vi "Set Fill Color.vi"(8 "error in (no error)":errorcluster, 9 "Color":u32(colorbox), 10 "Shape refnum":refnum<k7>) -> (0 "error out":errorcluster, 2 "reference out":refnum<k7>)   [LabVIEW 2020, in "lvpptx.lvlib"]
uses:
  lvpptx.lvlib
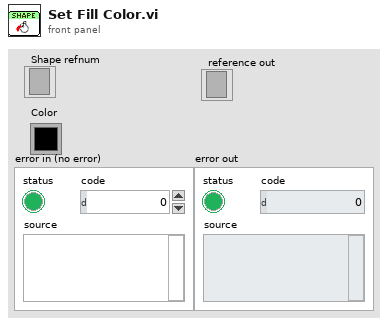
[diagram p1: front panel]
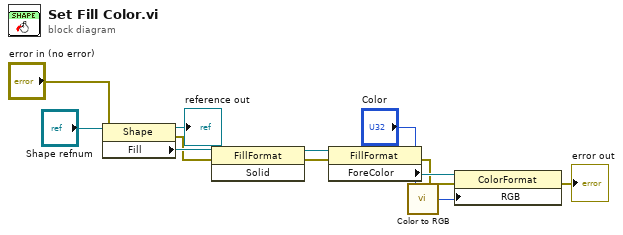
[diagram p0: block diagram]
diagram:
  n1 = property class="Shape"(reference="Shape refnum", error in="error in (no error)") -> (reference out=→"reference out":refnum<k7>, error out=w3:errorcluster, "Fill"=w11:refnum<k7>)
  n2 = invoke class="FillFormat" method="Solid"(reference=w11, error in=w3) -> (reference out=w10:refnum<k7>, error out=w9:errorcluster)  [unwired: 1 in, 1 out]
  n3 = property class="FillFormat"(reference=w10, error in=w9) -> (error out=w2:errorcluster, "ForeColor"=w8:refnum<k7>)  [unwired: 1 out]
  n4 = call "Color to RGB.vi"("Color"="Color") -> ("32bit out"=w7:u32)  [unwired: 4 in]
  n5 = property class="ColorFormat"(reference=w8, error in=w2, "RGB"=w7) -> (error out=→"error out":errorcluster)  [unwired: 1 out]
